vi "libssh2_version.vi"(8 "error in (no error)":errorcluster, 10 "required_version (0 = any)":i32) -> (0 "error out":errorcluster, 2 "version":string)   [LabVIEW 2013, in "libssh2.lvlib"]
doc: "Get the version of libssh2."
uses:
  libssh2.lvlib
  Global Settings.vi
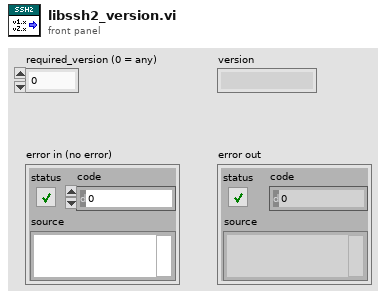
[diagram p1: front panel]
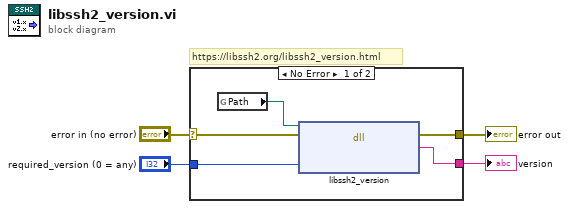
[diagram p0: block diagram]
diagram:
  # "https://libssh2.org/libssh2_version.html"
  n1 = case shown="No Error" "error in (no error)" {
    selector: "error in (no error)" -> [w5 w10]
    tunnel: [w8 w10] -> w4
    tunnel: "required_version (0 = any)" -> [w7 _]
    tunnel: [w6 _] -> w2
    frame No Error {
      n2 = global read "Global Settings.vi" "Path"() -> (w9:path)
      n3 = dll-call lib="?" fn="libssh2_version"(path in=w9, error in=w5, "required_version"=w7) -> (error out=w8:errorcluster, "return value"=w6:string)  [unwired: 2 in, 1 out]
    }
    frame Error {
    }
  }
  "error out" <- w4
  "version" <- w2
